vi "SQLite Edit Transaction Test.vi"(7 "Test DB Set Up Command":string, 8 "Error In (no error)":errorcluster, 11 "SQLite DB Operator In":refnum<class "SQLite DB Operator.lvclass">) -> (0 "Error Out":errorcluster, 3 "SQLite DB Operator Out":refnum<class "SQLite DB Operator.lvclass">)   [LabVIEW 2023]
uses:
  Clasess/SQLite DB Operator/SQLite DB Operator.lvclass
  Clasess/DB Records/Expenses Tracker Transaction/Public/Ctrls/Transaction.ctl
  Clasess/DB Records/Expenses Tracker Transaction/Expenses Tracker Transaction.lvclass
  H:/Desktop/LabVIEW/LabView Repo/Expenses-Tracker-DB-Operator/Interfaces/Expenses Tracker Record/Expenses Tracker Record.lvclass
  Support/Editing/Edit Record Assert Error.vi
  Support/Editing/Edit Record Assert Not Error.vi
  <vilib>/drjdpowell/SQLite Library/SQL Connection/Execute SQL (1D Cluster).vi
  <vilib>/addons/_JKI Toolkits/Caraya/classes/Test/Test.lvclass
  <vilib>/drjdpowell/SQLite Library/SQLite.lvlib
  H:/Desktop/LabVIEW/LabView Repo/Expenses-Tracker-DB-Operator/Clasess/DB Records/Expenses Tracker Transaction/Expenses Tracker Transaction.lvclass
  <vilib>/drjdpowell/SQLite Library/SQL Connection/Connection.lvclass
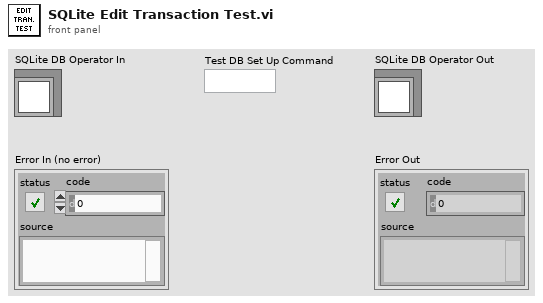
[diagram p1: front panel]
types:
  T1 = typedef "Expenses Tracker Transaction.lvclass/Transaction.ctl" = cluster{"ID":u32, "Name":string, "Is_income":bool, "Value":dbl, "Amount":dbl, "Total":dbl, "Date_of_entry":timestamp, "Date_of_occurence":timestamp, "Last_update":timestamp, "Category":u32, "Subcategory":u32, "Cycle":u32, "Description":string}
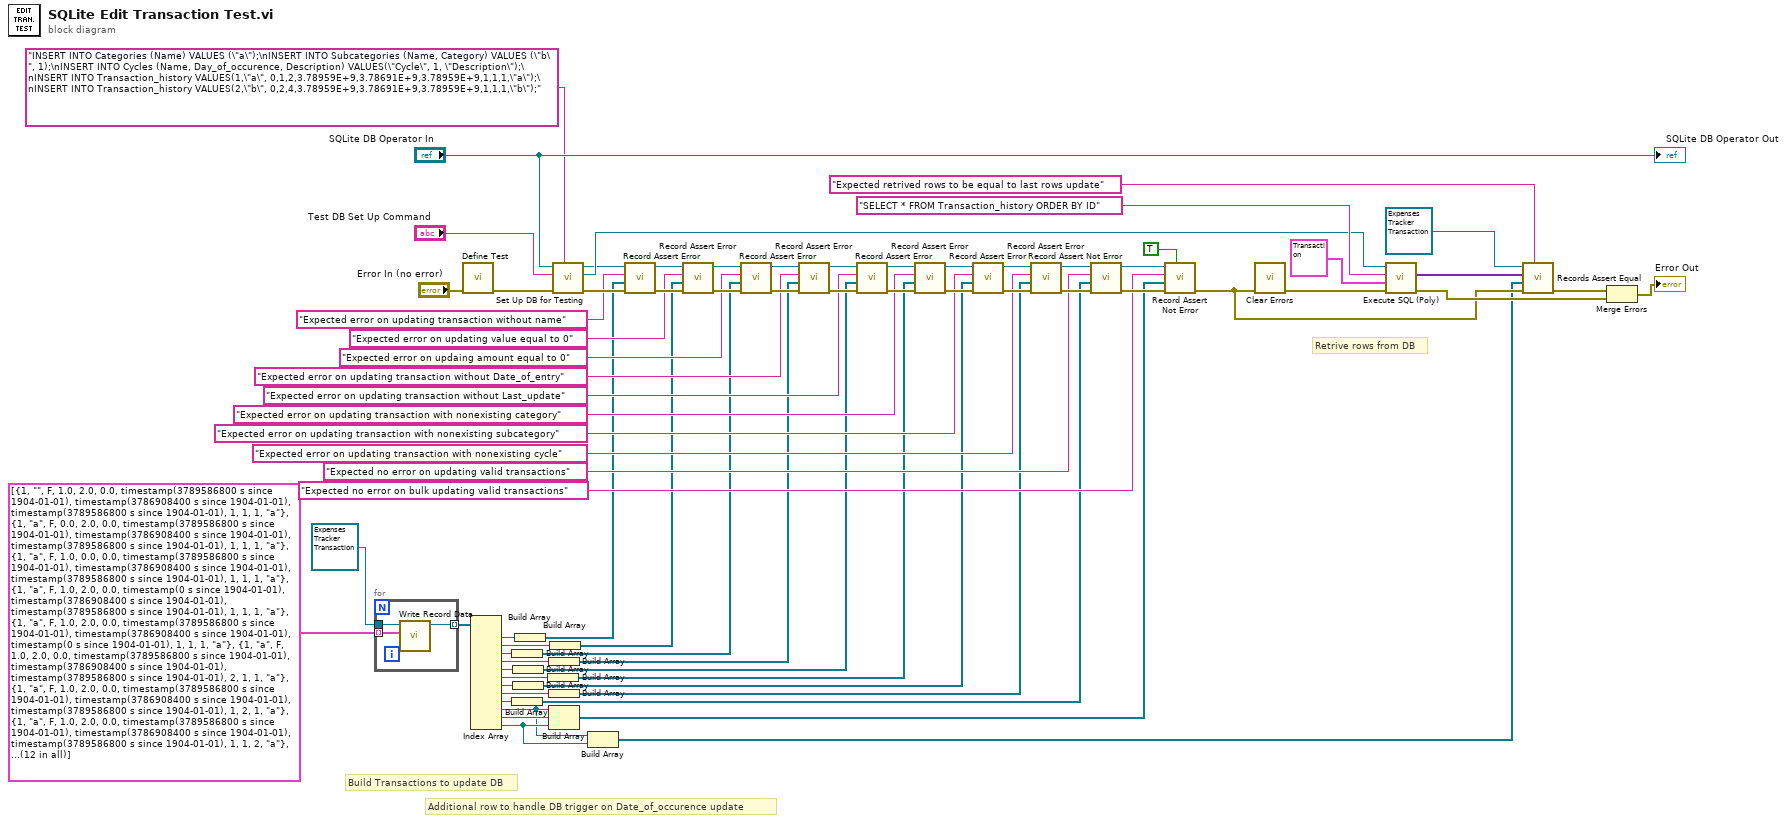
[diagram p0: block diagram]
diagram:
  # "Additional row to handle DB trigger on Date_of_occurence update"
  # "Retrive rows from DB"
  # "Build Transactions to update DB"
  n1 = for {
    tunnel: T1[] [{"ID"=1, "Name"="", "Is_income"=FALSE, "Value"=1.0, "Amount"=2.0, "Total"=0.0, "Date_of_entry"=timestamp(3789586800 s since 1904-01-01), "Date_of_occurence"=timestamp(3786908400 s since 1904-01-01), "Last_update"=timestamp(3789586800 s since 1904-01-01), "Category"=1, "Subcategory"=1, "Cycle"=1, "Description"="a"}, {"ID"=1, "Name"="a", "Is_income"=FALSE, "Value"=0.0, "Amount"=2.0, "Total"=0.0, "Date_of_entry"=timestamp(3789586800 s since 1904-01-01), "Date_of_occurence"=timestamp(3786908400 s since 1904-01-01), "Last_update"=timestamp(3789586800 s since 1904-01-01), "Category"=1, "Subcategory"=1, "Cycle"=1, "Description"="a"}, {"ID"=1, "Name"="a", "Is_income"=FALSE, "Value"=1.0, "Amount"=0.0, "Total"=0.0, "Date_of_entry"=timestamp(3789586800 s since 1904-01-01), "Date_of_occurence"=timestamp(3786908400 s since 1904-01-01), "Last_update"=timestamp(3789586800 s since 1904-01-01), "Category"=1, "Subcategory"=1, "Cycle"=1, "Description"="a"}, {"ID"=1, "Name"="a", "Is_income"=FALSE, "Value"=1.0, "Amount"=2.0, "Total"=0.0, "Date_of_entry"=timestamp(0 s since 1904-01-01), "Date_of_occurence"=timestamp(3786908400 s since 1904-01-01), "Last_update"=timestamp(3789586800 s since 1904-01-01), "Category"=1, "Subcategory"=1, "Cycle"=1, "Description"="a"}, {"ID"=1, "Name"="a", "Is_income"=FALSE, "Value"=1.0, "Amount"=2.0, "Total"=0.0, "Date_of_entry"=timestamp(3789586800 s since 1904-01-01), "Date_of_occurence"=timestamp(3786908400 s since 1904-01-01), "Last_update"=timestamp(0 s since 1904-01-01), "Category"=1, "Subcategory"=1, "Cycle"=1, "Description"="a"}, {"ID"=1, "Name"="a", "Is_income"=FALSE, "Value"=1.0, "Amount"=2.0, "Total"=0.0, "Date_of_entry"=timestamp(3789586800 s since 1904-01-01), "Date_of_occurence"=timestamp(3786908400 s since 1904-01-01), "Last_update"=timestamp(3789586800 s since 1904-01-01), "Category"=2, "Subcategory"=1, "Cycle"=1, "Description"="a"}, {"ID"=1, "Name"="a", "Is_income"=FALSE, "Value"=1.0, "Amount"=2.0, "Total"=0.0, "Date_of_entry"=timestamp(3789586800 s since 1904-01-01), "Date_of_occurence"=timestamp(3786908400 s since 1904-01-01), "Last_update"=timestamp(3789586800 s since 1904-01-01), "Category"=1, "Subcategory"=2, "Cycle"=1, "Description"="a"}, {"ID"=1, "Name"="a", "Is_income"=FALSE, "Value"=1.0, "Amount"=2.0, "Total"=0.0, "Date_of_entry"=timestamp(3789586800 s since 1904-01-01), "Date_of_occurence"=timestamp(3786908400 s since 1904-01-01), "Last_update"=timestamp(3789586800 s since 1904-01-01), "Category"=1, "Subcategory"=1, "Cycle"=2, "Description"="a"}, {"ID"=1, "Name"="e", "Is_income"=FALSE, "Value"=1.0, "Amount"=2.0, "Total"=0.0, "Date_of_entry"=timestamp(3789586800 s since 1904-01-01), "Date_of_occurence"=timestamp(3786908400 s since 1904-01-01), "Last_update"=timestamp(3789586800 s since 1904-01-01), "Category"=1, "Subcategory"=1, "Cycle"=1, "Description"="a"}, {"ID"=1, "Name"="f", "Is_income"=FALSE, "Value"=1.0, "Amount"=2.0, "Total"=2.0, "Date_of_entry"=timestamp(3789586800 s since 1904-01-01), "Date_of_occurence"=timestamp(3786908400 s since 1904-01-01), "Last_update"=timestamp(3789586800 s since 1904-01-01), "Category"=1, "Subcategory"=1, "Cycle"=1, "Description"="a"}, {"ID"=2, "Name"="g", "Is_income"=FALSE, "Value"=2.0, "Amount"=4.0, "Total"=8.0, "Date_of_entry"=timestamp(3789586800 s since 1904-01-01), "Date_of_occurence"=timestamp(0 s since 1904-01-01), "Last_update"=timestamp(3792092400 s since 1904-01-01), "Category"=1, "Subcategory"=1, "Cycle"=1, "Description"="b"}, {"ID"=2, "Name"="g", "Is_income"=FALSE, "Value"=2.0, "Amount"=4.0, "Total"=8.0, "Date_of_entry"=timestamp(3789586800 s since 1904-01-01), "Date_of_occurence"=timestamp(3789586800 s since 1904-01-01), "Last_update"=timestamp(3792092400 s since 1904-01-01), "Category"=1, "Subcategory"=1, "Cycle"=1, "Description"="b"}] ("Array") -> [w76] mode=indexing
    tunnel: refnum<class "Expenses Tracker Transaction.lvclass"> refnum ("Expenses Tracker Category") -> [w75]
    tunnel: [w74] -> w70 mode=indexing
    n2 = call-dynamic "Write Record Data.vi"("Record"=w76, "Expenses Tracker Transaction In"=w75) -> ("Expenses Tracker Transaction Out"=w74:refnum<class "Expenses Tracker Transaction.lvclass">)  [unwired: 8 in, 1 out]
  }
  n3 = call <vilib>:"Define Test.vi"("error in (no error)"="Error In (no error)") -> ("error out"=w63:errorcluster)  [unwired: 9 in, 1 out]
  n4 = Index Array(array=w70) -> (element #1=w24:refnum<class "Expenses Tracker Transaction.lvclass">, element #2=w22:refnum<class "Expenses Tracker Transaction.lvclass">, element #3=w20:refnum<class "Expenses Tracker Transaction.lvclass">, element #4=w18:refnum<class "Expenses Tracker Transaction.lvclass">, element #5=w16:refnum<class "Expenses Tracker Transaction.lvclass">, element #6=w14:refnum<class "Expenses Tracker Transaction.lvclass">, element #7=w12:refnum<class "Expenses Tracker Transaction.lvclass">, element #8=w10:refnum<class "Expenses Tracker Transaction.lvclass">, element #9=w8:refnum<class "Expenses Tracker Transaction.lvclass">, element #10=w2:refnum<class "Expenses Tracker Transaction.lvclass">, element #11=w6:refnum<class "Expenses Tracker Transaction.lvclass">, element #12=w3:refnum<class "Expenses Tracker Transaction.lvclass">)  [unwired: 12 in]
  n5 = Build Array(w20) -> (w19:refnum<class "Expenses Tracker Transaction.lvclass">[])
  n6 = Build Array(w8) -> (w7:refnum<class "Expenses Tracker Transaction.lvclass">[])
  n7 = Build Array(w16) -> (w15:refnum<class "Expenses Tracker Transaction.lvclass">[])
  n8 = Build Array(w12) -> (w11:refnum<class "Expenses Tracker Transaction.lvclass">[])
  n9 = Build Array(w24) -> (w23:refnum<class "Expenses Tracker Transaction.lvclass">[])
  n10 = Build Array(w14) -> (w13:refnum<class "Expenses Tracker Transaction.lvclass">[])
  n11 = Build Array(w18) -> (w17:refnum<class "Expenses Tracker Transaction.lvclass">[])
  n12 = Build Array(w10) -> (w9:refnum<class "Expenses Tracker Transaction.lvclass">[])
  n13 = Build Array(w2, w6, w3) -> (w4:refnum<class "Expenses Tracker Transaction.lvclass">[])
  n14 = Build Array(w22) -> (w21:refnum<class "Expenses Tracker Transaction.lvclass">[])
  n15 = call "Set Up DB for Testing.vi"("Additional Set Up Commands"="INSERT INTO Categories (Name) VALUES (\"a\");\nINSERT INTO Subcategories (Name, Category) VALUES (\"b\", 1);\nINSERT INTO Cycles (Name, Day_of_occurence, Description) VALUES(\"Cycle\", 1, \"Description\");\nINSERT INTO Transaction_history VALUES(1,\"a\", 0,1,2,3.78959E+9,3.78691E+9,3.78959E+9,1,1,1,\"a\");\nINSERT INTO Transaction_history VALUES(2,\"b\", 0,2,4,3.78959E+9,3.78691E+9,3.78959E+9,1,1,1,\"b\");", "Error In (no error)"=w63, "Test DB Set Up Command"="Test DB Set Up Command", "SQLite DB Operator In"="SQLite DB Operator In") -> ("Error Out"=w43:errorcluster, "SQLite Connection"=w67:refnum<class "Connection.lvclass">, "SQLite DB Operator Out"=w40:refnum<class "SQLite DB Operator.lvclass">)  [unwired: 5 in]
  n16 = Build Array(w2, w3) -> (w1:refnum<class "Expenses Tracker Transaction.lvclass">[])
  n17 = call-poly "Record Assert Error.vi"("Error In"=w43, "Records"=w23, "Assertion Label"="Expected error on updating transaction without name" ("Label (VI Title)"), "SQLite DB Operator In"=w40) -> ("Error Out"=w52:errorcluster, "SQLite DB Operator Out"=w53:refnum<class "SQLite DB Operator.lvclass">)  [unwired: 6 in]
  n18 = call-poly "Record Assert Error.vi"("Error In"=w52, "Records"=w21, "Assertion Label"="Expected error on updating value equal to 0" ("Label (VI Title)"), "SQLite DB Operator In"=w53) -> ("Error Out"=w50:errorcluster, "SQLite DB Operator Out"=w51:refnum<class "SQLite DB Operator.lvclass">)  [unwired: 6 in]
  n19 = call-poly "Record Assert Error.vi"("Error In"=w50, "Records"=w19, "Assertion Label"="Expected error on updaing amount equal to 0" ("Label (VI Title)"), "SQLite DB Operator In"=w51) -> ("Error Out"=w57:errorcluster, "SQLite DB Operator Out"=w56:refnum<class "SQLite DB Operator.lvclass">)  [unwired: 6 in]
  n20 = call-poly "Record Assert Error.vi"("Error In"=w57, "Records"=w17, "Assertion Label"="Expected error on updating transaction without Date_of_entry" ("Label (VI Title)"), "SQLite DB Operator In"=w56) -> ("Error Out"=w48:errorcluster, "SQLite DB Operator Out"=w49:refnum<class "SQLite DB Operator.lvclass">)  [unwired: 6 in]
  n21 = call-poly "Record Assert Error.vi"("Error In"=w48, "Records"=w15, "Assertion Label"="Expected error on updating transaction without Last_update" ("Label (VI Title)"), "SQLite DB Operator In"=w49) -> ("Error Out"=w46:errorcluster, "SQLite DB Operator Out"=w47:refnum<class "SQLite DB Operator.lvclass">)  [unwired: 6 in]
  n22 = call-poly "Record Assert Error.vi"("Error In"=w46, "Records"=w13, "Assertion Label"="Expected error on updating transaction with nonexisting category" ("Label (VI Title)"), "SQLite DB Operator In"=w47) -> ("Error Out"=w44:errorcluster, "SQLite DB Operator Out"=w45:refnum<class "SQLite DB Operator.lvclass">)  [unwired: 6 in]
  n23 = call-poly "Record Assert Error.vi"("Error In"=w44, "Records"=w11, "Assertion Label"="Expected error on updating transaction with nonexisting subcategory" ("Label (VI Title)"), "SQLite DB Operator In"=w45) -> ("Error Out"=w54:errorcluster, "SQLite DB Operator Out"=w55:refnum<class "SQLite DB Operator.lvclass">)  [unwired: 6 in]
  n24 = call-poly "Record Assert Error.vi"("Error In"=w54, "Records"=w9, "Assertion Label"="Expected error on updating transaction with nonexisting cycle" ("Label (VI Title)"), "SQLite DB Operator In"=w55) -> ("Error Out"=w42:errorcluster, "SQLite DB Operator Out"=w41:refnum<class "SQLite DB Operator.lvclass">)  [unwired: 6 in]
  n25 = call-poly "Record Assert Not Error.vi"("Error In"=w42, "Records"=w7, "Assertion Label"="Expected no error on updating valid transactions" ("Label (VI Title)"), "SQLite DB Operator In"=w41) -> ("Error Out"=w28:errorcluster, "SQLite DB Operator Out"=w27:refnum<class "SQLite DB Operator.lvclass">)  [unwired: 6 in]
  n26 = call-poly "Record Assert Not Error.vi"("Bulk Update?"=TRUE, "Error In"=w28, "Records"=w4, "Assertion Label"="Expected no error on bulk updating valid transactions" ("Label (VI Title)"), "SQLite DB Operator In"=w27) -> ("Error Out"=w25:errorcluster)  [unwired: 5 in, 1 out]
  n27 = call <vilib>:"Clear Errors.vi"("error in (no error)"=w25) -> ("error out"=w58:errorcluster)  [unwired: 5 in, 1 out]
  n28 = call-poly <vilib>:"Execute SQL (Poly).vi"("error in (no error)"=w58, "Cluster (or Array of Clusters)"=T1 {"ID"=0, "Name"="", "Is_income"=FALSE, "Value"=0.0, "Amount"=0.0, "Total"=0.0, "Date_of_entry"=timestamp(0 s since 1904-01-01), "Date_of_occurence"=timestamp(0 s since 1904-01-01), "Last_update"=timestamp(0 s since 1904-01-01), "Category"=0, "Subcategory"=0, "Cycle"=0, "Description"=""} ("Transaction"), "SQL"="SELECT * FROM Transaction_history ORDER BY ID", "SQLite Connection in"=w67) -> ("error out"=w59:errorcluster, "Result Set (Array of Clusters)"=w30:variant[])  [unwired: 5 in, 1 out]
  n29 = call "Records Assert Equal.vi"("Assertion Label"="Expected retrived rows to be equal to last rows update" ("Label (VI Title)"), "Error In"=w25, "Correct Records"=w1, "Typedef Records"=w30, "Expenses Tracker Record In"=refnum<class "Expenses Tracker Transaction.lvclass"> refnum ("Expenses Tracker Category")) -> ("Error Out"=w60:errorcluster)  [unwired: 6 in]
  n30 = Merge Errors(w60, w59) -> (→"Error Out":errorcluster)
  "SQLite DB Operator Out" <- "SQLite DB Operator In"
